vi "BUFFERload.vi"(8 "Error In (no error)":errorcluster, 11 "ICImagingControl In":refnum<k7>) -> (0 "Error Out":errorcluster, 1 "Image Out":T1, 2 "SampleStartTime":dbl, 3 "ICImagingControl Out":refnum<k7>, 4 "SampleEndTime":dbl)   [LabVIEW 2018]
uses:
  <vilib>/vision/Image Controls.llb/IMAQ Image.ctl
  C:/Program Files (x86)/National Instruments/LabVIEW 2018/user.lib/IC LabVIEW Extension 2_64.dll
panel:
  in  "BorderSize":i32=3
  out "imaq_ptr":u32
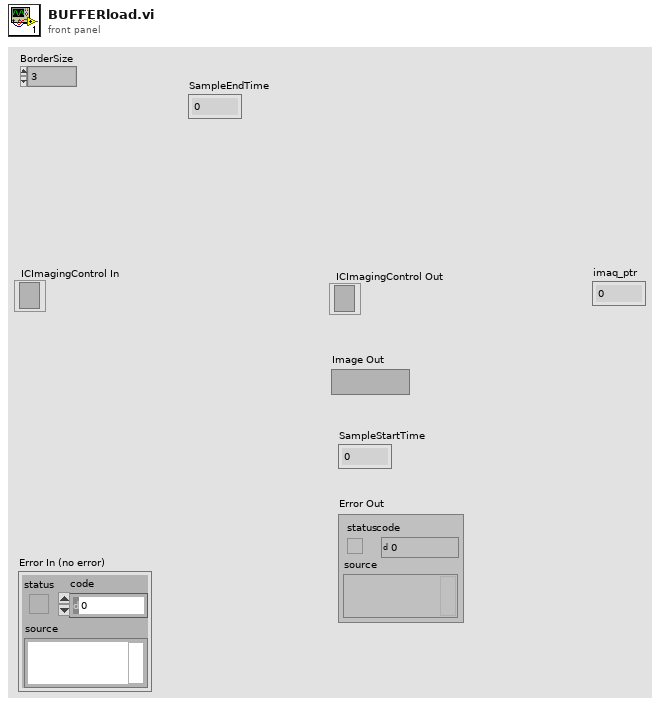
[diagram p1: front panel]
types:
  T1 = typedef "IMAQ Image.ctl" = refnum<image>
  T2 = typedef "Image Type" = u32
  T3 = enum32{"Map Pixel Pointer", "Unmap Pixel Pointer", "Get Pixels Infos"}
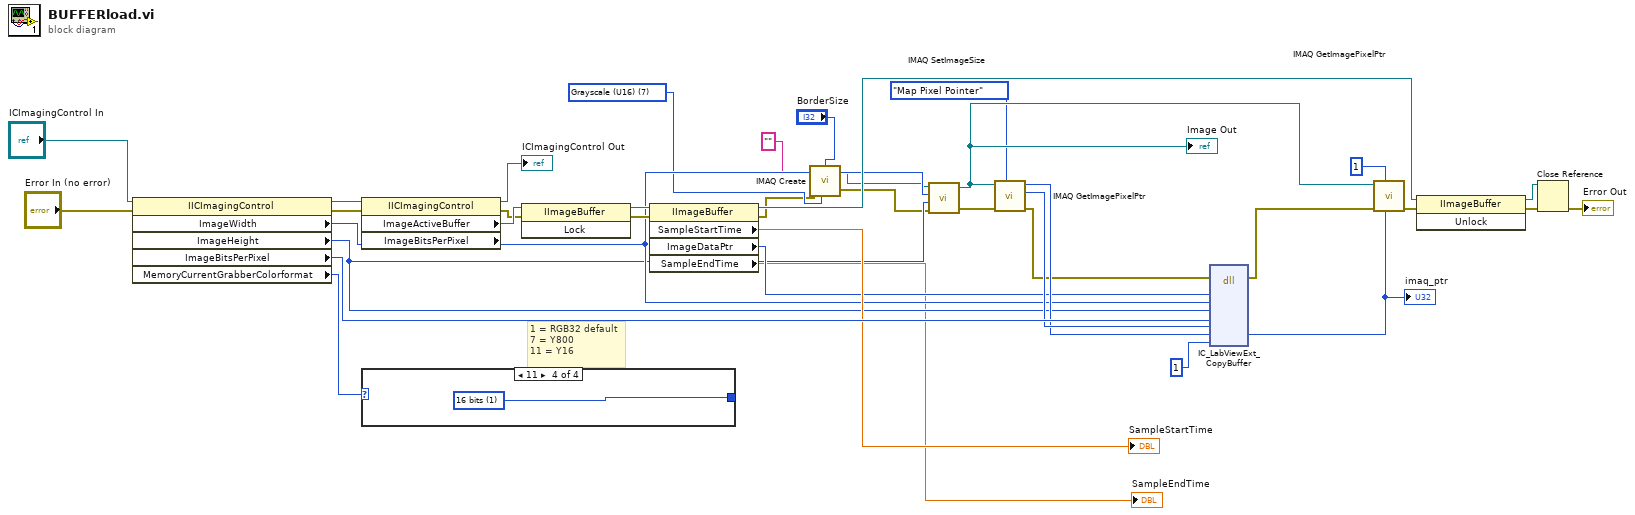
[diagram p0: block diagram]
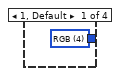
[diagram p2: hidden frame]
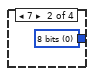
[diagram p3: hidden frame]
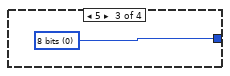
[diagram p4: hidden frame]
diagram:
  w6 = T2 7 items=["Grayscale (U8)", "Grayscale (I16)", "Grayscale (SGL)", "Complex (CSG)", "RGB (U32)", "HSL (U32)", "RGB (U64)", "Grayscale (U16)"] ("Image Type")
  # "1 = RGB32 default\n7 = Y800\n11 = Y16"
  n1 = property class="IICImagingControl"(reference="ICImagingControl In", error in="Error In (no error)") -> (reference out=w19:refnum<k7>, error out=w15:errorcluster, "ImageWidth"=w11:i32, "ImageHeight"=w10:i32, "ImageBitsPerPixel"=w33:i32, "MemoryCurrentGrabberColorformat"=w20:i32)
  n2 = property class="IICImagingControl" props=["ImageActiveBuffer", "ImageBitsPerPixel"](reference=w19, error in=w15) -> (reference out=→"ICImagingControl Out":refnum<k7>, error out=w16:errorcluster, "ImageActiveBuffer"=w18:refnum<k7>)  [unwired: 1 out]
  n3 = case shown="11" w20 {
    tunnel: [w38 w39 w40 w41] -> _
    frame 1, Default {
      w38 = u32 4 items=["8 bits", "16 bits", "Float", "Complex", "RGB", "HSL"] ("Image Type")
    }
    frame 7 {
      w39 = u32 0 items=["8 bits", "16 bits", "Float", "Complex", "RGB", "HSL"] ("Image Type")
    }
    frame 5 {
      w40 = u32 0 items=["8 bits", "16 bits", "Float", "Complex", "RGB", "HSL"] ("Image Type")
    }
    frame 11 {
      w41 = u32 1 items=["8 bits", "16 bits", "Float", "Complex", "RGB", "HSL"] ("Image Type")
    }
  }
  n4 = invoke class="IImageBuffer" method="Lock"(reference=w18, error in=w16) -> (reference out=w21:refnum<k7>, error out=w22:errorcluster)  [unwired: 1 in, 1 out]
  n5 = property class="IImageBuffer"(reference=w21, error in=w22) -> (reference out=w23:refnum<k7>, error out=w4:errorcluster, "SampleStartTime"=→"SampleStartTime":dbl, "ImageDataPtr"=w14:i64, "SampleEndTime"=→"SampleEndTime":dbl)
  n6 = call "IMAQ Create"("Border Size"="BorderSize", "Image Name"="", "Image Type"=w6, "error in (no error)"=w4) -> ("New Image"=w5:T1, "error out"=w3:errorcluster)  [unwired: 1 in]
  n7 = call "IMAQ SetImageSize"("error in (no error)"=w3, "Y Resolution"=w10, "X Resolution"=w11, "Image"=w5) -> ("error out"=w35:errorcluster, "Image Out"=w36:T1)  [unwired: 1 in]
  "Image Out" <- w36
  n8 = call "IMAQ GetImagePixelPtr"("Function"=T3."Map Pixel Pointer", "error in (no error)"=w35, "Image"=w36) -> ("error out"=w2:errorcluster, "LineWidth(Pixels)"=w32:i32, "Pixel Pointer out"=w31:u64)  [unwired: 3 in, 3 out]
  n9 = dll-call lib="C:/Program Files (x86)/National Instruments/LabVIEW 2018/user.lib/IC LabVIEW Extension 2_64.dll" fn="IC_LabViewExt_CopyBuffer"(error in=w2, "data"=w14, "width"=w11, "height"=w10, "bpp"=w33, "imaq_width"=w32, "imaq_ptr"=w31, "bFlip"=u8 1) -> (error out=w1:errorcluster, "imaq_ptr"=w30:u64)  [unwired: 9 in, 1 out]
  "imaq_ptr" <- w30
  n10 = call "IMAQ GetImagePixelPtr"("Pixel Pointer in"=w30, "Function"=1, "error in (no error)"=w1, "Image"=w36) -> ("error out"=w27:errorcluster)  [unwired: 2 in, 5 out]
  n11 = invoke class="IImageBuffer" method="Unlock"(reference=w23, error in=w27) -> (reference out=w26:refnum<k7>, error out=w25:errorcluster)  [unwired: 1 in, 1 out]
  n12 = Close Reference(reference=w26, error in (no error)=w25) -> (error out=→"Error Out":errorcluster)
